vi "NET_DriveRPM.vi"(8 "Read(F) Write(T)":bool, 10 "Right RPM In":dbl, 11 "Left RPM In":dbl) -> (2 "Right RPM Out":dbl, 3 "Left RPM Out":dbl)   [LabVIEW 2017]
uses:
  <vilib>/Rock Robotics/Network Tables/NT Read Numeric Array.vi
  <vilib>/Rock Robotics/Network Tables/NT Write Numeric Array.vi
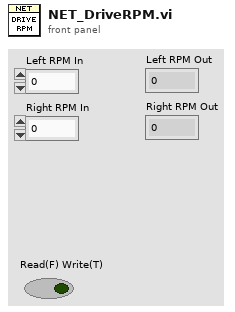
[diagram p1: front panel]
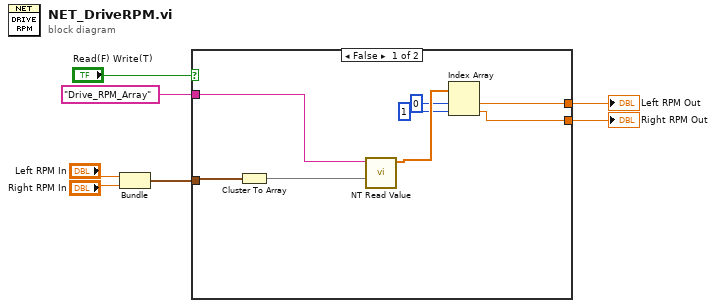
[diagram p0: block diagram]
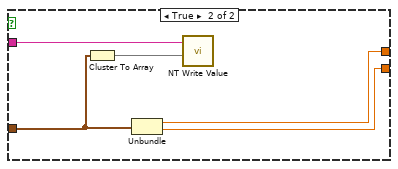
[diagram p2: hidden frame]
diagram:
  n1 = Bundle("Left RPM In"="Left RPM In", "Right RPM In"="Right RPM In") -> (w3:cluster{"Left RPM In":dbl, "Right RPM In":dbl})  [unwired: 1 in]
  n2 = case shown="False" "Read(F) Write(T)" {
    tunnel: w3 -> [w14 w18]
    tunnel: "Drive_RPM_Array" ("Name") -> [w15 w19]
    tunnel: [w9 w17] -> w2
    tunnel: [w8 w16] -> w1
    frame False {
      n3 = Cluster To Array(cluster=w14) -> (array=w13:dbl[])
      n4 = call-poly <vilib>:"NT Read Value.vi"("Default Value"=w13, "Name"=w15) -> ("Numeric Array"=w12:dbl[])  [unwired: 8 in, 1 out]
      n5 = Index Array(array=w12, index #1=0 ("index"), index #2=1 ("index")) -> (element #1=w9:dbl, element #2=w8:dbl)
    }
    frame True {
      n6 = Cluster To Array(cluster=w18) -> (array=w20:dbl[])
      n7 = Unbundle(w18) -> ("Left RPM In"=w17:dbl, "Right RPM In"=w16:dbl)
      n8 = call-poly <vilib>:"NT Write Value.vi"("Numeric Array"=w20, "Name"=w19) -> ()  [unwired: 9 in, 1 out]
    }
  }
  "Left RPM Out" <- w2
  "Right RPM Out" <- w1
